vi "BK Precision 8500B Series Run Peak Test.vi"() -> ()   [LabVIEW 2019]
doc: "Exemplifies monitoring the Min/Max Voltage and Min/Max Current in the mode selected."
uses:
  <instrlib>/BK Precision 8500B Series/BK Precision 8500B Series.lvlib
panel:
  out "Min Peak Voltage":dbl format="%_6f"
  out "Min Peak Current":dbl format="%_6f"
  out "Max Peak Current":dbl format="%_6f"
  out "Max Peak Voltage":dbl format="%_6f"
  in  "?":bool
  in  "Operation Mode":u16(ring) items=["CC", "CV", "CR", "CW"]
  in  "VISA resource name":refnum<visa-resource-name>
  in  "Serial Configuration":cluster{"Baud Rate":u32}={"Baud Rate"=9600} {"Baud Rate" items=["300"=300, "600"=600, "1200"=1200, "2400"=2400, "4800"=4800, "9600"=9600, "19200"=19200]}
  # "(c) 2019 B&K Precision Corporation.  ALL RIGHTS RESERVED."
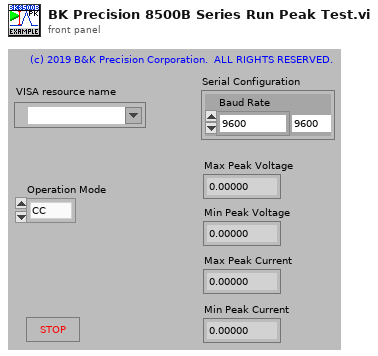
[diagram p1: front panel]
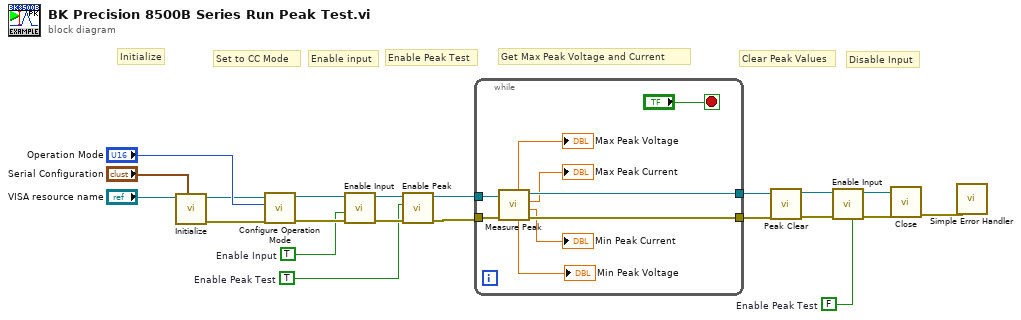
[diagram p0: block diagram]
diagram:
  w4 = TRUE  # Enable Input
  w5 = FALSE  # Enable Peak Test
  w6 = TRUE  # Enable Peak Test
  # "Get Max Peak Voltage and Current"
  # "Disable Input"
  # "Clear Peak Values"
  # "Enable input"
  # "Enable Peak Test"
  # "Set to CC Mode"
  # "Initialize"
  n1 = call <instrlib>:"Initialize.vi"("Serial Configuration"="Serial Configuration", "VISA resource name"="VISA resource name") -> ("error out"=w17:errorcluster, "VISA resource name out"=w18:refnum<visa-resource-name>)  [unwired: 8 in]
  n2 = call <instrlib>:"Configure Operation Mode.vi"("error in (no error)"=w17, "Operation Mode (0:CC)"="Operation Mode", "VISA resource name"=w18) -> ("error out"=w15:errorcluster, "VISA resource name out"=w16:refnum<visa-resource-name>)  [unwired: 7 in]
  n3 = call <instrlib>:"Enable Input.vi"("error in (no error)"=w15, "Enable Input (F: False)"=w4, "VISA resource name"=w16) -> ("error out"=w14:errorcluster, "VISA resource name out"=w13:refnum<visa-resource-name>)  [unwired: 7 in]
  n4 = call <instrlib>:"Enable Peak.vi"("error in (no error)"=w14, "Enable Peak Test (F: False)"=w6, "VISA resource name"=w13) -> ("error out"=w11:errorcluster, "VISA resource name out"=w12:refnum<visa-resource-name>)  [unwired: 7 in]
  n5 = while {
    tunnel: [w27] -> w10
    tunnel: [w26] -> w9
    tunnel: w11 -> [w29]
    tunnel: w12 -> [w28]
    stop <- "?" stop-if-true
    n6 = call <instrlib>:"Measure Peak.vi"("error in (no error)"=w29, "VISA resource name"=w28) -> ("error out"=w26:errorcluster, "Min Peak Current"=→"Min Peak Current":dbl, "Max Peak Current"=→"Max Peak Current":dbl, "VISA resource name out"=w27:refnum<visa-resource-name>, "Min Peak Voltage"=→"Min Peak Voltage":dbl, "Max Peak Voltage"=→"Max Peak Voltage":dbl)  [unwired: 4 in]
  }
  n7 = call <instrlib>:"Peak Clear.vi"("error in (no error)"=w9, "VISA resource name"=w10) -> ("error out"=w7:errorcluster, "VISA resource name out"=w8:refnum<visa-resource-name>)  [unwired: 8 in]
  n8 = call <instrlib>:"Enable Input.vi"("error in (no error)"=w7, "Enable Input (F: False)"=w5, "VISA resource name"=w8) -> ("error out"=w2:errorcluster, "VISA resource name out"=w3:refnum<visa-resource-name>)  [unwired: 7 in]
  n9 = call <instrlib>:"Close.vi"("error in (no error)"=w2, "VISA resource name"=w3) -> ("error out"=w1:errorcluster)  [unwired: 9 in]
  n10 = call <vilib>:"Simple Error Handler.vi"("error in (no error)"=w1) -> ()  [unwired: 4 in, 5 out]
